vi "ex4-5.vi"() -> ()   [LabVIEW 2009]
uses:
  <vilib>/NXT/Dual Mode Library/Sound/PlayC.vi
  <vilib>/NXT/Dual Mode Library/Waits/Wait_Num.vi
  <vilib>/NXT/Dual Mode Library/Motors/MotorOn.vi
panel:
  out "Numeric":dbl
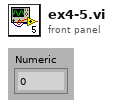
[diagram p1: front panel]
types:
  T1 = typedef "LVHSConnector.ctl" = cluster{"error":errorcluster, "address":string, "NXT #":i32, "Show Error":bool, "Connection":u16}
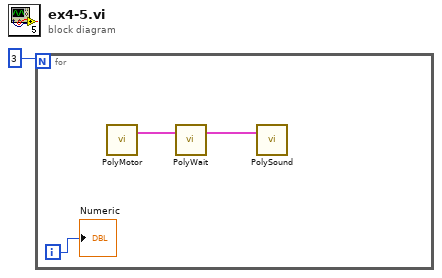
[diagram p0: block diagram]
diagram:
  n1 = for {
    N: 3 -> [_]
    i -> [w2]
    n2 = call-poly <vilib>:"PolyMotor.vi"() -> ("NXT"=w4:T1)  [unwired: 4 in]
    n3 = call-poly <vilib>:"PolyWait.vi"("NXT"=w4) -> ("NXT"=w3:T1)  [unwired: 3 in]
    n4 = call-poly <vilib>:"PolySound.vi"("NXT"=w3) -> ()  [unwired: 3 in, 1 out]
    "Numeric" <- w2
  }
